vi "Create VI From Template For Oneof Class.vi"(8 "error in (no error)":errorcluster, 9 "VI name":string, 10 "template name":string, 11 "LVClassLibrary in":refnum<vi>) -> (0 "error out":errorcluster, 3 "saved VI path":path)   [LabVIEW 2019, in "gRPC Template Creation Utility.lvlib"]
uses:
  gRPC Template Creation Utility.lvlib
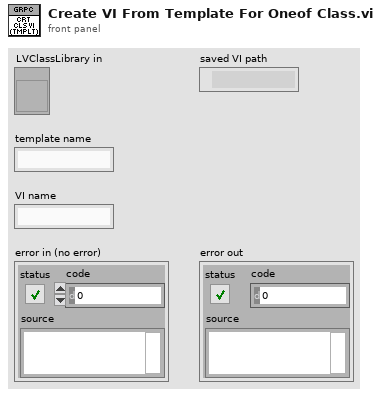
[diagram p1: front panel]
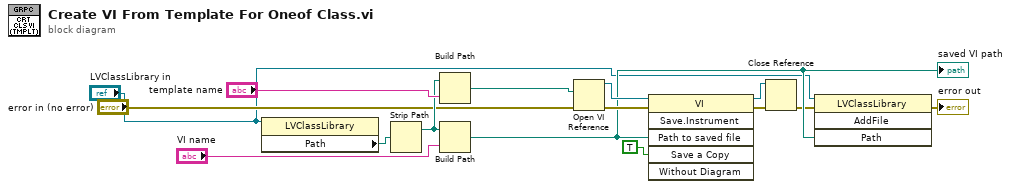
[diagram p0: block diagram]
diagram:
  n1 = property class="LVClassLibrary"(reference="LVClassLibrary in") -> ("Path"=w3:path)  [unwired: 1 in, 2 out]
  n2 = Strip Path(path=w3) -> (stripped path=w4:path)  [unwired: 1 out]
  n3 = Build Path(base path=w4, name or relative path="template name") -> (appended path=w10:path)
  n4 = Build Path(base path=w4, name or relative path="VI name") -> (appended path=w9:path)
  "saved VI path" <- w9
  n5 = Open VI Reference(vi path=w10, error in (no error)="error in (no error)") -> (vi reference=w12:refnum<vi>, error out=w11:errorcluster)  [unwired: 4 in]
  n6 = invoke class="VI" method="Save.Instrument"(reference=w12, error in=w11, "Path to saved file"=w9, "Save a Copy"=TRUE) -> (reference out=w15:refnum<vi>, error out=w14:errorcluster)  [unwired: 2 in, 4 out]
  n7 = Close Reference(reference=w15, error in (no error)=w14) -> (error out=w6:errorcluster)
  n8 = invoke class="LVClassLibrary" method="AddFile"(reference="LVClassLibrary in", error in=w6, "Path"=w9) -> (error out=→"error out":errorcluster)  [unwired: 1 in, 3 out]
